vi "Get Pin Names from Expanded Pin Information.vi"(0 "Expanded Pin Information":T1[](array[typedef])) -> (4 "Pins":tag[](array[tag]))   [LabVIEW 2019]
uses:
  TSM Expanded Pin Information.ctl
  TSM Pin Type Identifier.ctl
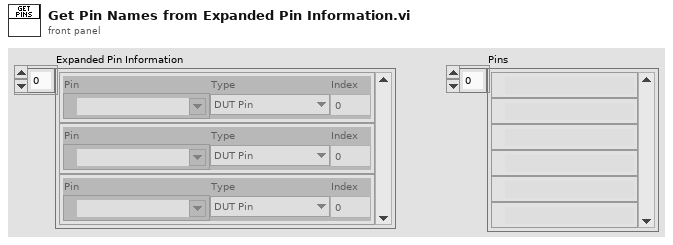
[diagram p1: front panel]
types:
  T1 = typedef "TSM Expanded Pin Information.ctl" = cluster{"Pin":tag, "Type":T2, "Index":i32}
  T2 = typedef "TSM Pin Type Identifier.ctl" = enum8{"DUT Pin", "System Pin", "Pin Group", "Not Determined"}
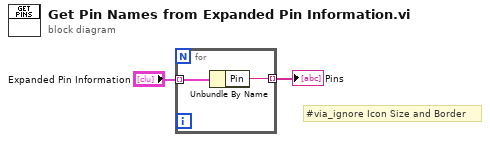
[diagram p0: block diagram]
diagram:
  # "#via_ignore Icon Size and Border"
  n1 = for {
    tunnel: "Expanded Pin Information" -> [w4] mode=indexing
    tunnel: [w3] -> w1 mode=indexing
    n2 = Unbundle By Name(w4) -> ("Pin"=w3:tag)
  }
  "Pins" <- w1
